vi "Create.vi"(8 "error in (no error)":errorcluster, 10 "Show Receive?":bool) -> (0 "error out":errorcluster, 3 "Filter by Process out":refnum<class "Filter by Is Receive.lvclass">)   [LabVIEW 2020, in "Filter by Is Receive.lvclass"]
uses:
  Filter by Is Receive.lvclass
  Filter by Is Receive.lvclass/Filter by Is Receive.ctl
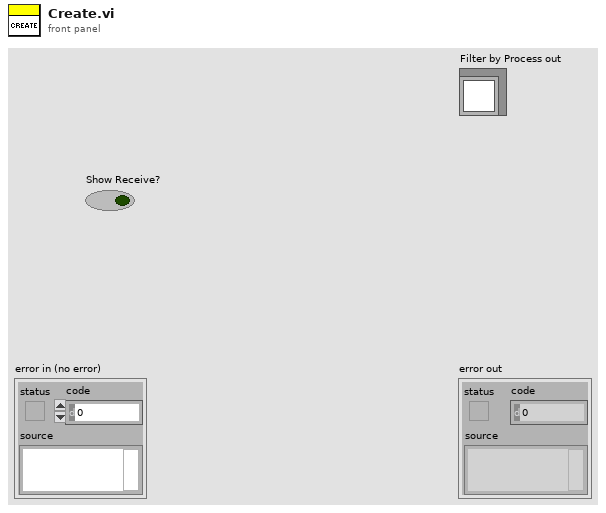
[diagram p1: front panel]
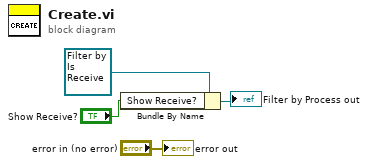
[diagram p0: block diagram]
diagram:
  n1 = Bundle By Name(cluster=refnum<class "Filter by Is Receive.lvclass"> refnum ("Filter by Process out"), "Show Receive?"="Show Receive?") -> (→"Filter by Process out":refnum<class "Filter by Is Receive.lvclass">)
  "error out" <- "error in (no error)"
